vi "DIO 20-bit.vi"(0 "DIO 0 Refnum":refnum<k21>="ConnectorA/DIO0", 1 "DIO 1 Refnum":refnum<k21>="ConnectorA/DIO1", 2 "DIO 2 Refnum":refnum<k21>="ConnectorA/DIO2", 3 "DIO 3 Refnum":refnum<k21>="ConnectorA/DIO3", 4 "DIO 4 Refnum":refnum<k21>="ConnectorA/DIO4", 5 "DIO 5 Refnum":refnum<k21>="ConnectorA/DIO5", 6 "DIO 6 Refnum":refnum<k21>="ConnectorA/DIO6", 7 "DIO 7 Refnum":refnum<k21>="ConnectorA/DIO7", 8 "DIO 8 Refnum":refnum<k21>="ConnectorA/DIO8", 9 "DIO 9 Refnum":refnum<k21>="ConnectorA/DIO8", 10 "DIO 10 Refnum":refnum<k21>="ConnectorA/DIO10", 11 "DIO 11 Refnum":refnum<k21>="ConnectorA/DIO11", 12 "DIO 12 Refnum":refnum<k21>="ConnectorA/DIO12", 13 "DIO 13 Refnum":refnum<k21>="ConnectorA/DIO13", 14 "DIO 14 Refnum":refnum<k21>="ConnectorA/DIO14", 15 "DIO 15 Refnum":refnum<k21>="ConnectorA/DIO15", 16 "DIO 16 Refnum":refnum<k21>="ConnectorA/DIO16", 17 "DIO 17 Refnum":refnum<k21>="ConnectorA/DIO17", 18 "DIO 18 Refnum":refnum<k21>="ConnectorA/DIO18", 19 "DIO 19 Refnum":refnum<k21>="ConnectorA/DIO19", 20 "OUT 19:0":fxp<+,20,20> format="%08b", 21 "DIR 19:0":fxp<+,20,20> format="%08b") -> (22 "IN 19:0":fxp<+,20,20> format="%08b")   [LabVIEW 2019]
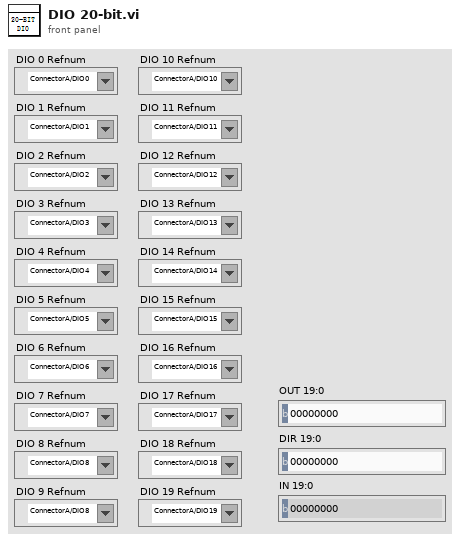
[diagram p1: front panel]
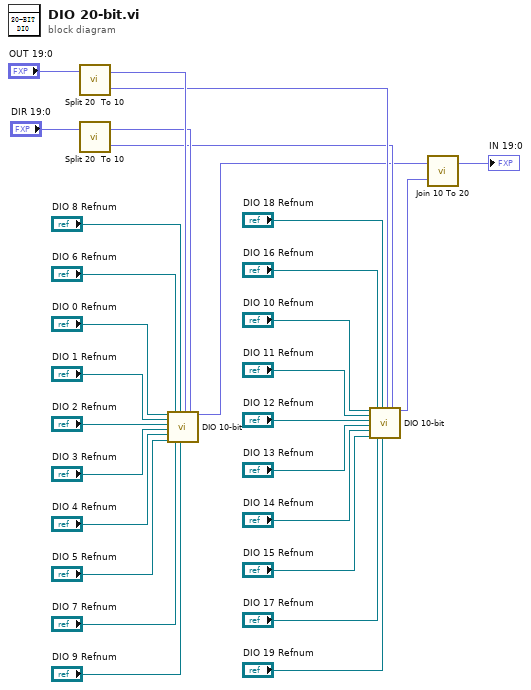
[diagram p0: block diagram]
diagram:
  n1 = call "Split 20  To 10.vi"("IN 19:0"="OUT 19:0") -> ("OUT 19:10"=w6:fxp<+,10,10>, "OUT 9:0"=w7:fxp<+,10,10>)  [unwired: 1 in]
  n2 = call "Split 20  To 10.vi"("IN 19:0"="DIR 19:0") -> ("OUT 19:10"=w4:fxp<+,10,10>, "OUT 9:0"=w5:fxp<+,10,10>)  [unwired: 1 in]
  n3 = call "DIO 10-bit.vi"("DIO 0 Refnum"="DIO 0 Refnum", "DIO 1 Refnum"="DIO 1 Refnum", "DIO 2 Refnum"="DIO 2 Refnum", "DIO 3 Refnum"="DIO 3 Refnum", "DIO 4 Refnum"="DIO 4 Refnum", "DIO 5 Refnum"="DIO 5 Refnum", "DIO 6 Refnum"="DIO 6 Refnum", "DIO 7 Refnum"="DIO 7 Refnum", "DIO 8 Refnum"="DIO 8 Refnum", "DIO 9 Refnum"="DIO 9 Refnum", "OUT 9:0"=w7, "DIR 9:0"=w5) -> ("IN 9:0"=w3:fxp<+,10,10>)  [unwired: 7 in]
  n4 = call "DIO 10-bit.vi"("DIO 0 Refnum"="DIO 10 Refnum", "DIO 1 Refnum"="DIO 11 Refnum", "DIO 2 Refnum"="DIO 12 Refnum", "DIO 3 Refnum"="DIO 13 Refnum", "DIO 4 Refnum"="DIO 14 Refnum", "DIO 5 Refnum"="DIO 15 Refnum", "DIO 6 Refnum"="DIO 16 Refnum", "DIO 7 Refnum"="DIO 17 Refnum", "DIO 8 Refnum"="DIO 18 Refnum", "DIO 9 Refnum"="DIO 19 Refnum", "OUT 9:0"=w6, "DIR 9:0"=w4) -> ("IN 9:0"=w2:fxp<+,10,10>)  [unwired: 7 in]
  n5 = call "Join 10 To 20.vi"("IN 19:10"=w2, "IN 9:0"=w3) -> ("OUT 19:0"=→"IN 19:0":fxp<+,20,20>)  [unwired: 1 in]
